vi "configure BMC.vi"(8 "error in (no error)":errorcluster, 11 "BMC in":refnum<class "BMC.lvclass">) -> (0 "error out":errorcluster, 3 "BMC out":refnum<class "BMC.lvclass">)   [LabVIEW 2012, in "BMC.lvclass"]
uses:
  BMC.lvclass
  BMC.lvclass/BMC.ctl
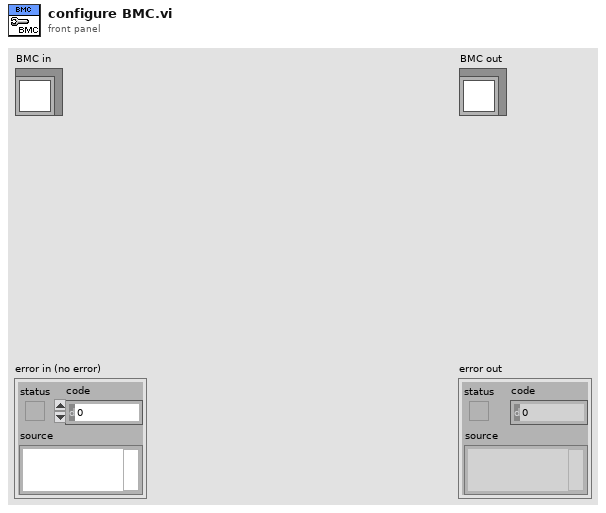
[diagram p1: front panel]
types:
  T1 = enum16{"CIUsb_CONTROL_ASSERT_FRAME_SYNC", "CIUsb_CONTROL_DEASSERT_FRAME_SYNC", "CIUsb_CONTROL_ASSERT_FRESET", "CIUsb_CONTROL_DEASSERT_FRESET", "CIUsb_CONTROL_ASSERT_HV_ENAB", "CIUsb_CONTROL_DEASSERT_HV_ENAB", "CIUsb_CONTROL_ASSERT_LV_SHDN", "CIUsb_CONTROL_DEASSERT_LV_SHDN", "CIUsb_CONTROL_ASSERT_EXT_I2C", "CIUsb_CONTROL_DEASSERT_EXT_I2C", "CIUsb_CONTROL_MINI_MODE"}
  T2 = enum32{"CIUsb_CONTROL_ASSERT_FRAME_SYNC", "CIUsb_CONTROL_DEASSERT_FRAME_SYNC", "CIUsb_CONTROL_ASSERT_FRESET", "CIUsb_CONTROL_DEASSERT_FRESET", "CIUsb_CONTROL_ASSERT_HV_ENAB", "CIUsb_CONTROL_DEASSERT_HV_ENAB", "CIUsb_CONTROL_ASSERT_LV_SHDN", "CIUsb_CONTROL_DEASSERT_LV_SHDN", "CIUsb_CONTROL_ASSERT_EXT_I2C", "CIUsb_CONTROL_DEASSERT_EXT_I2C", "CIUsb_CONTROL_MINI_MODE"}
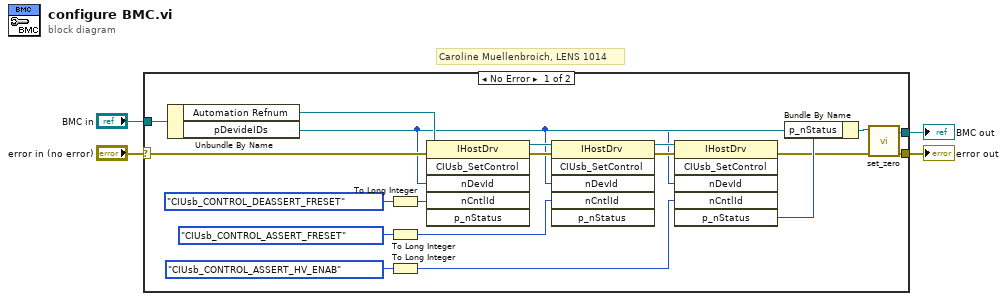
[diagram p0: block diagram]
diagram:
  # "Caroline Muellenbroich, LENS 1014"
  n1 = case shown="No Error" "error in (no error)" {
    selector: "error in (no error)" -> [w23 w25]
    tunnel: [w8 w25] -> w3
    tunnel: [w5 w24] -> w1
    tunnel: "BMC in" -> [w18 w24]
    frame No Error {
      n2 = Unbundle By Name(w18) -> ("Automation Refnum"=w20:refnum<k7>, "pDevideIDs"=w10:i32)
      n3 = To Long Integer(number=T2."CIUsb_CONTROL_DEASSERT_FRESET") -> (32bit integer=w14:i32)
      n4 = To Long Integer(number=T1."CIUsb_CONTROL_ASSERT_FRESET") -> (32bit integer=w12:i32)
      n5 = To Long Integer(number=T1."CIUsb_CONTROL_ASSERT_HV_ENAB") -> (32bit integer=w9:i32)
      n6 = invoke class="IHostDrv" method="CIUsb_SetControl"(reference=w20, error in=w23, "nDevId"=w10, "nCntlId"=w14) -> (reference out=w19:refnum<k7>, error out=w22:errorcluster)  [unwired: 2 in, 4 out]
      n7 = invoke class="IHostDrv" method="CIUsb_SetControl"(reference=w19, error in=w22, "nDevId"=w10, "nCntlId"=w12) -> (reference out=w16:refnum<k7>, error out=w21:errorcluster)  [unwired: 2 in, 4 out]
      n8 = invoke class="IHostDrv" method="CIUsb_SetControl"(reference=w16, error in=w21, "nDevId"=w10, "nCntlId"=w9) -> (error out=w7:errorcluster, "p_nStatus"=w17:i32)  [unwired: 2 in, 4 out]
      n9 = Bundle By Name(cluster=w18, "p_nStatus"=w17) -> (w6:refnum<class "BMC.lvclass">)
      n10 = call-dynamic "set_zero.vi"("error in (no error)"=w7, "BMC in"=w6) -> ("error out"=w8:errorcluster, "BMC out"=w5:refnum<class "BMC.lvclass">)  [unwired: 8 in]
    }
    frame Error {
    }
  }
  "error out" <- w3
  "BMC out" <- w1
